vi "HEWH Process Header Names.vi"(9 "Search Expression 2":string, 10 "Search Expression 1":string, 11 "Header":string[](array[string])) -> (3 "Output Header":string[](array[string]))   [LabVIEW 2023]
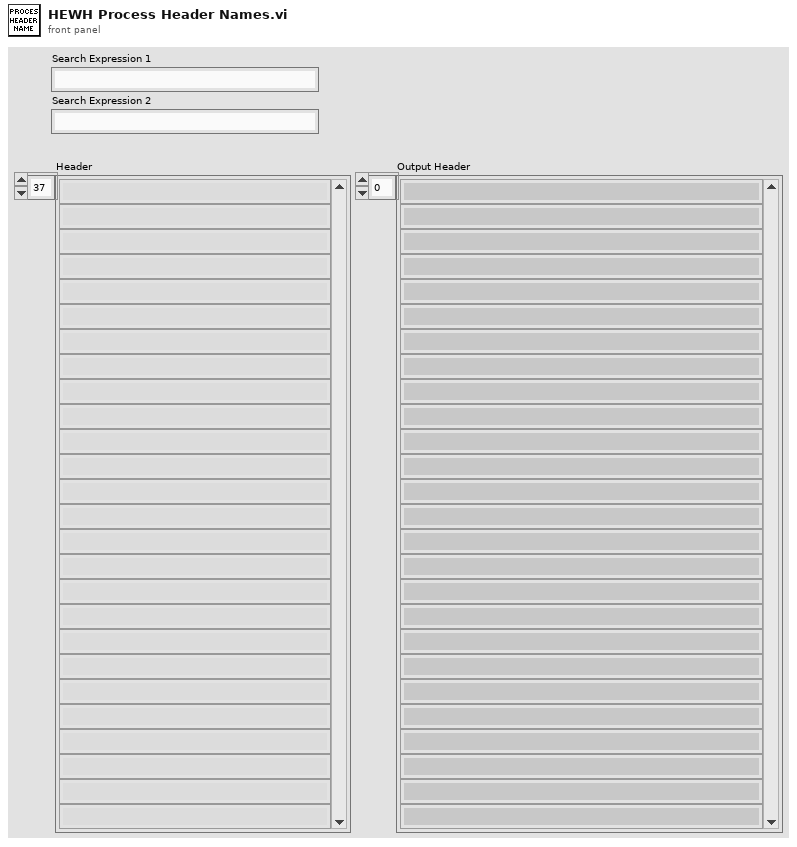
[diagram p1: front panel]
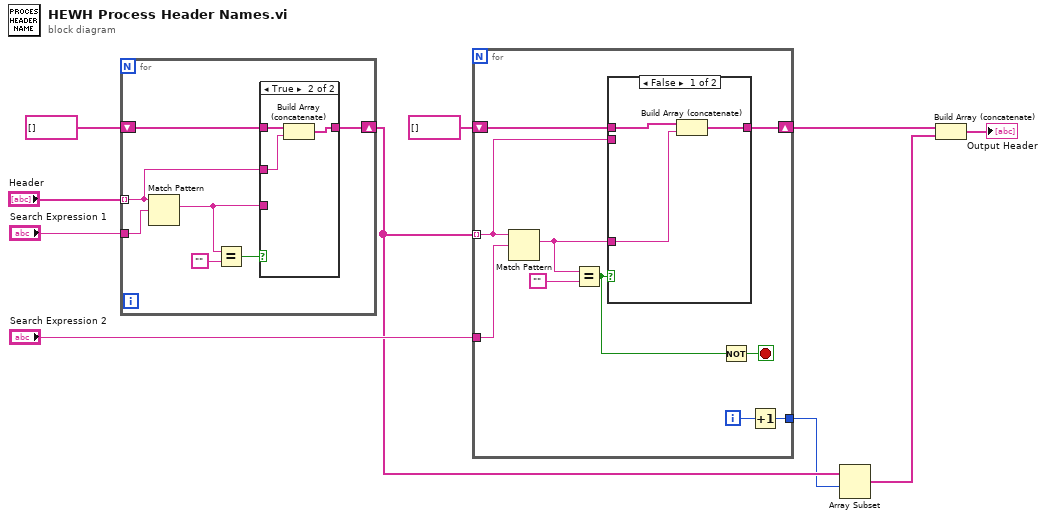
[diagram p0: block diagram]
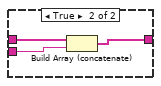
[diagram p2: hidden frame]
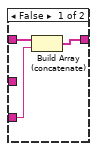
[diagram p3: hidden frame]
diagram:
  n1 = for {
    tunnel: "Header" -> [w11] mode=indexing
    tunnel: "Search Expression 1" -> [w17]
    shift-right: [w15] -> w5
    shift-left: string[] [] -> [w16]
    n2 = Match Pattern(string=w11, regular expression=w17) -> (match substring=w14:string)  [unwired: 1 in, 3 out]
    n3 = Equal?(x=w14, y="") -> (x = y?=w12:bool)
    n4 = case shown="True" w12 {
      tunnel: w16 -> [w20 w23]
      tunnel: w14 -> [w19 _]
      tunnel: [w18 w21] -> w15
      tunnel: w11 -> [_ w22]
      frame False {
        n5 = Build Array (concatenate)(w20, w19) -> (w18:string[])
      }
      frame True {
        n6 = Build Array (concatenate)(w23, w22) -> (w21:string[])
      }
    }
  }
  n7 = for {
    tunnel: w5 -> [w28] mode=indexing
    tunnel: "Search Expression 2" -> [w33]
    shift-right: [w31] -> w3
    shift-left: string[] [] -> [w32]
    tunnel: [w24] -> w4
    i -> [w25]
    stop <- w27 stop-if-true
    n8 = Match Pattern(string=w28, regular expression=w33) -> (match substring=w30:string)  [unwired: 1 in, 3 out]
    n9 = Equal?(x=w30, y="") -> (x = y?=w26:bool)
    n10 = case shown="False" w26 {
      tunnel: w32 -> [w36 w39]
      tunnel: w30 -> [w35 _]
      tunnel: [w34 w38] -> w31
      tunnel: w28 -> [_ w37]
      frame False {
        n11 = Build Array (concatenate)(w36, w35) -> (w34:string[])
      }
      frame True {
        n12 = Build Array (concatenate)(w39, w37) -> (w38:string[])
      }
    }
    n13 = Not(x=w26) -> (.not. x?=w27:bool)
    n14 = Increment(x=w25) -> (x+1=w24:i32)
  }
  n15 = Array Subset(array=w5, index=w4) -> (w2:string[])  [unwired: 1 in]
  n16 = Build Array (concatenate)(w3, w2) -> (→"Output Header":string[])
